vi "General - Generate Error if True.vi"(5 "Generate Error":bool, 6 "error in (no error)":errorcluster, 8 "String":string, 9 "Error (-1000)":i32=-1000) -> (0 "error out":errorcluster)   [LabVIEW 2020]
doc: "If \"Generate Error\" is true then an error is created and passed to \"error out\".\n\nIf \"error in\" indicates an error condition then it is passed to \"error out\" ignoring any other inputs."
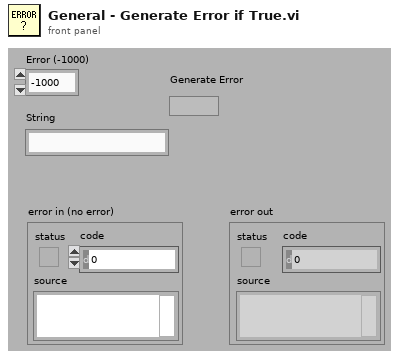
[diagram p1: front panel]
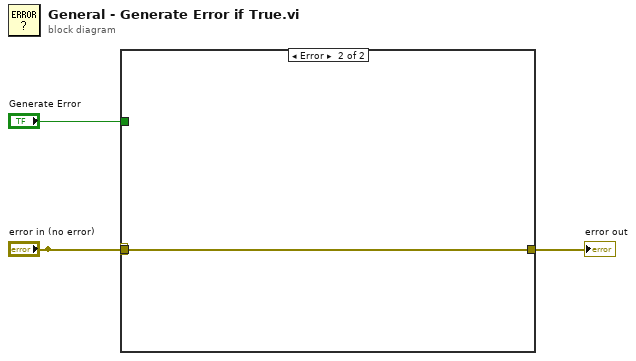
[diagram p0: block diagram]
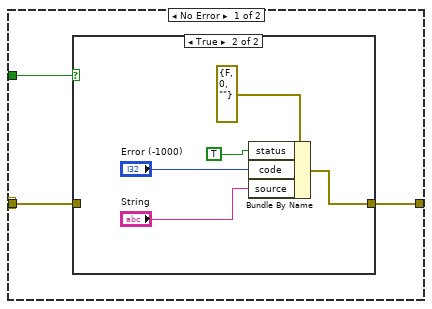
[diagram p2: hidden frame]
diagram:
  n1 = case shown="Error" "error in (no error)" {
    tunnel: "error in (no error)" -> [w5 w13]
    tunnel: [w4 w13] -> w3
    tunnel: "Generate Error" -> [w6 _]
    frame No Error {
      n2 = case shown="True" w6 {
        tunnel: w5 -> [w7 _]
        tunnel: [w7 w11] -> w4
        frame False {
        }
        frame True {
          n3 = Bundle By Name(cluster=errorcluster {"status"=FALSE, "code"=0, "source"=""} ("error out"), "status"=TRUE, "code"="Error (-1000)", "source"="String") -> (w11:errorcluster)
        }
      }
    }
    frame Error {
    }
  }
  "error out" <- w3
